vi "display_slider.vi"(8 "error in":errorcluster, 11 "cluster refs in":T1) -> (0 "error out":errorcluster)   [LabVIEW 2011]
uses:
  type_definitions/clusters/controls_refs.ctl
  global_variables.vi
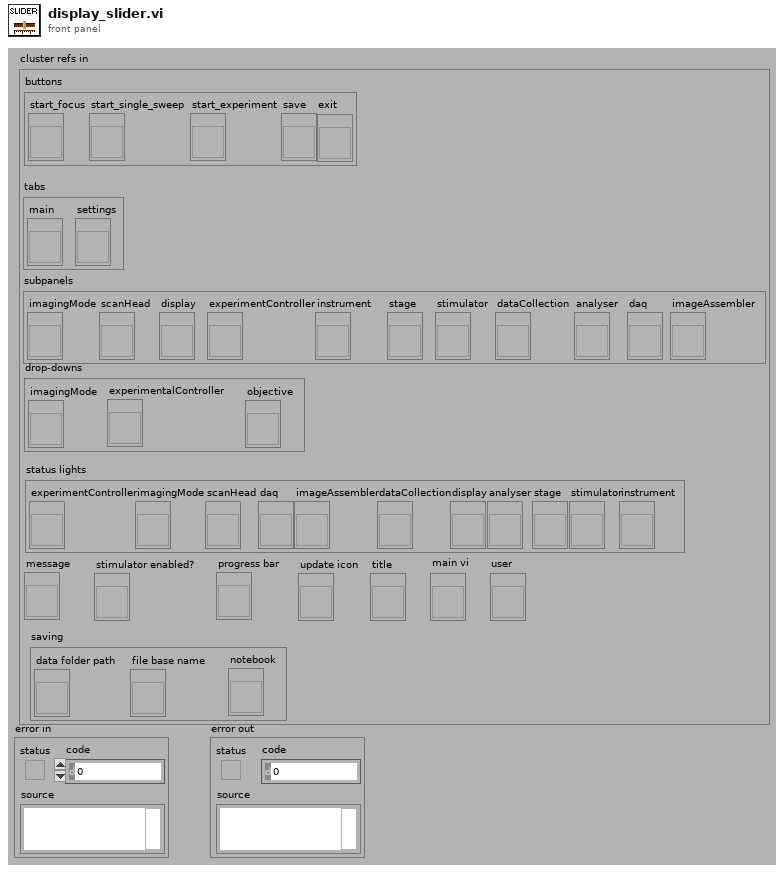
[diagram p1: front panel]
types:
  T1 = typedef "controls_refs.ctl" = cluster{"buttons":cluster{"start_focus":refnum<vi>, "start_single_sweep":refnum<vi>, "start_experiment":refnum<vi>, "save":refnum<vi>, "exit":refnum<vi>}, "tabs":cluster{"main":refnum<vi>, "settings":refnum<vi>}, "subpanels":cluster{"imagingMode":refnum<vi>, "scanHead":refnum<vi>, "display":refnum<vi>, "experimentController":refnum<vi>, "instrument":refnum<vi>, "stage":refnum<vi>, "stimulator":refnum<vi>, "dataCollection":refnum<vi>, "analyser":refnum<vi>, "daq":refnum<vi>, "imageAssembler":refnum<vi>}, "drop-downs":cluster{"imagingMode":refnum<vi>, "experimentalController":refnum<vi>, "objective":refnum<vi>}, "status lights":cluster{"experimentController":refnum<vi>, "imagingMode":refnum<vi>, "scanHead":refnum<vi>, "daq":refnum<vi>, "imageAssembler":refnum<vi>, "dataCollection":refnum<vi>, "display":refnum<vi>, "analyser":refnum<vi>, "stage":refnum<vi>, "stimulator":refnum<vi>, "instrument":refnum<vi>}, "message":refnum<vi>, "stimulator enabled?":refnum<vi>, "saving":cluster{"data folder path":refnum<vi>, "file base name":refnum<vi>, "notebook":refnum<vi>}, "progress bar":refnum<vi>, "update icon":refnum<vi>, "title":refnum<vi>, "main vi":refnum<vi>, "user":refnum<vi>}
  T2 = cluster{"experimentController":refnum<vi>, "imagingMode":refnum<vi>, "scanHead":refnum<vi>, "daq":refnum<vi>, "imageAssembler":refnum<vi>, "dataCollection":refnum<vi>, "display":refnum<vi>, "analyser":refnum<vi>, "stage":refnum<vi>, "stimulator":refnum<vi>, "instrument":refnum<vi>}
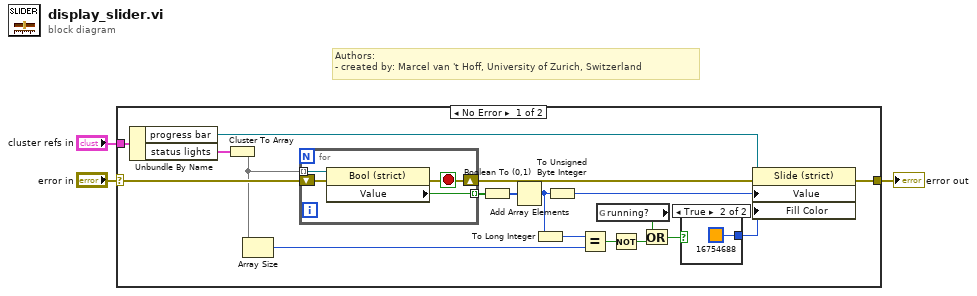
[diagram p0: block diagram]
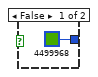
[diagram p2: hidden frame]
diagram:
  # "Authors: \n- created by: Marcel van 't Hoff, University of Zurich, Switzerland"
  n1 = case shown="No Error" "error in" {
    selector: "error in" -> [w21 w28]
    tunnel: [w19 w28] -> w3
    tunnel: "cluster refs in" -> [w20 _]
    frame No Error {
      n2 = Unbundle By Name(w20) -> ("progress bar"=w12:refnum<vi>, "status lights"=w18:T2)
      n3 = Cluster To Array(cluster=w18) -> (array=w17:refnum<vi>[])
      n4 = Array Size(array=w17) -> (size(s)=w7:i32)
      n5 = for {
        tunnel: [w25] -> w15 mode=indexing
        tunnel: w17 -> [w24] mode=indexing
        shift-right: [w27] -> w14
        shift-left: w21 -> [w26]
        stop <- w27 stop-if-true
        n6 = property class="Bool (strict)"(reference=w24, error in=w26) -> (error out=w27:errorcluster, "Value"=w25:bool)  [unwired: 1 out]
      }
      n7 = Boolean To (0,1)(Boolean=w15) -> (0, 1=w16:i16[])
      n8 = Add Array Elements(numeric array=w16) -> (sum=w6:i16)
      n9 = To Long Integer(number=w6) -> (32bit integer=w5:i32)
      n10 = To Unsigned Byte Integer(number=w6) -> (unsigned 8bit integer=w8:u8)
      n11 = Equal?(x=w5, y=w7) -> (x = y?=w4:bool)
      n12 = global read "global_variables.vi" "running?"() -> (w9:bool)
      n13 = Not(x=w4) -> (.not. x?=w11:bool)
      n14 = Or(x=w9, y=w11) -> (x .or. y?=w10:bool)
      n15 = case shown="True" w10 {
        tunnel: [u32 4499968 ("Color Box") u32 16754688 ("Color Box")] -> w13
        frame False {
        }
        frame True {
        }
      }
      n16 = property class="Slide (strict)"(reference=w12, error in=w14, "Value"=w8, "Fill Color"=w13) -> (error out=w19:errorcluster)  [unwired: 1 out]
    }
    frame Error {
    }
  }
  "error out" <- w3
